vi "Coord window-Add to picture-Sel coord.vi"(6 "Value":i32[](array[numeric]), 7 "Feature to draw":enum16{"Draw point", "Draw square"}(ring), 9 "ItemNames":string[][](array[string]), 10 "new picture in":picture, 11 "Picture map ref in":refnum<vi>) -> (2 "new picture out":picture, 3 "Picture map ref":refnum<vi>)   [LabVIEW 2020]
panel:
  in  "color":u32(colorbox)=60927
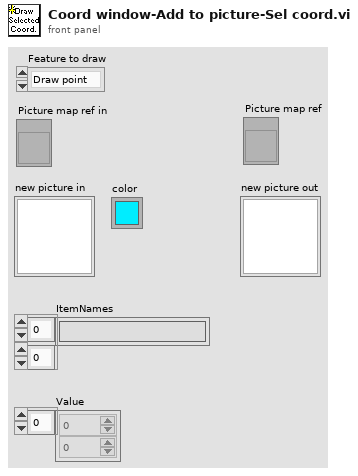
[diagram p1: front panel]
types:
  T1 = cluster{"Width":u16, "Style":enum32{"Solid", "Dash", "Dot", "DashDot", "DashDotDot"}}
  T2 = cluster{"Width":i16, "Style":enum32{"Solid", "Dash", "Dot", "DashDot", "DashDotDot"}}
  T3 = typedef "LVBoundsTypeDef.ctl" = cluster{"Width":u32, "Height":u32}
  T4 = cluster{"FOV/2-X (pixels)":i16, "FOV/2-Y (pixels)":i16}
  T5 = cluster{"left":i16, "top":i16, "right":i16, "bottom":i16}
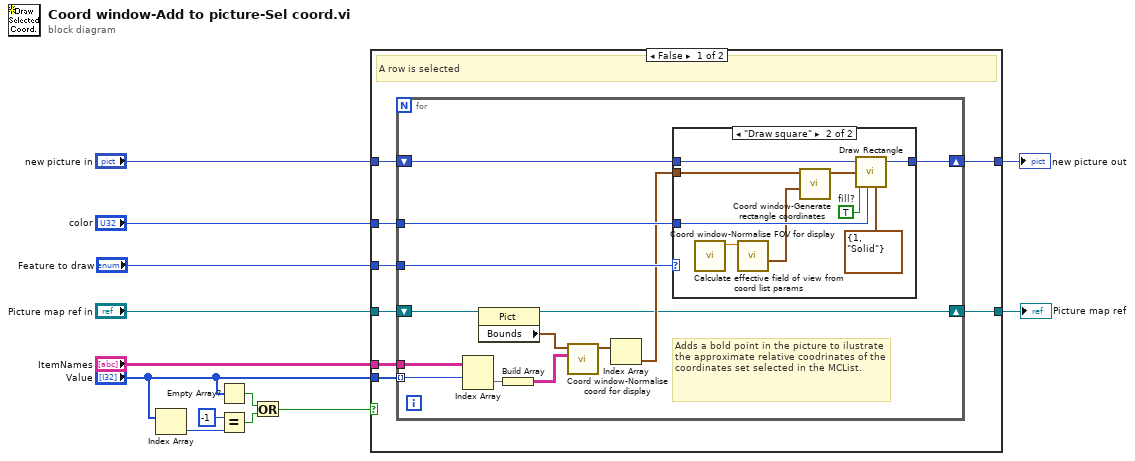
[diagram p0: block diagram]
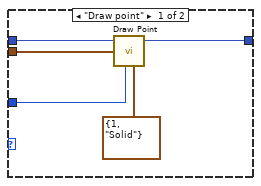
[diagram p2: hidden frame]
diagram:
  n1 = Index Array(array="Value") -> (element=w8:i32)  [unwired: 1 in]
  n2 = Empty Array?(array="Value") -> (empty?=w4:bool)
  n3 = Equal?(x=-1, y=w8) -> (x = y?=w5:bool)
  n4 = Or(x=w4, y=w5) -> (x .or. y?=w3:bool)
  n5 = case shown="False" w3 {
    tunnel: "new picture in" -> [w16 w50]
    tunnel: [w14 w50] -> w13
    tunnel: "Value" -> [w21 _]
    tunnel: "ItemNames" -> [w20 _]
    tunnel: "Picture map ref in" -> [w19 w49]
    tunnel: [w15 w49] -> w9
    tunnel: "color" -> [w17 _]
    tunnel: "Feature to draw" -> [w18 _]
    frame False {
      # "A row is selected"
      n6 = for {
        tunnel: w21 -> [w22] mode=indexing
        tunnel: w20 -> [w34]
        tunnel: w18 -> [w28]
        tunnel: w17 -> [w27]
        shift-right: [w24] -> w15
        shift-left: w19 -> [w30]
        shift-right: [w23] -> w14
        shift-left: w16 -> [w26]
        # "Adds a bold point in the picture to ilustrate the approximate relative coodrinates of the coordinates set selected in the MCList."
        n7 = Index Array(array=w34, index (row)=w22) -> (element=w33:string[])  [unwired: 1 in]
        n8 = property on="Property Node" class="Pict"(reference=w30) -> (reference out=w24:refnum<vi>, "Bounds"=w29:T3)  [unwired: 1 in, 1 out]
        n9 = Build Array(w33) -> (w32:string[][])
        n10 = call "Coord window-Normalise coord for display.vi"("MCList ItemNames"=w32, "Bounds"=w29) -> ("Normalised coordinates (for display)"=w31:cluster{"x":i16, "y":i16}[])  [unwired: 9 in]
        n11 = Index Array(array=w31) -> (element=w25:cluster{"x":i16, "y":i16})  [unwired: 1 in]
        n12 = case shown="\"Draw square\"" w28 {
          tunnel: w26 -> [w39 w48]
          tunnel: [w37 w47] -> w23
          tunnel: w25 -> [w36 w45]
          tunnel: w27 -> [w35 w46]
          frame "Draw point" {
            n13 = call <vilib>:"Draw Point.vi"("picture"=w39, "point(x,y)"=w36, "color(black)"=w35, "pen"=T1 {"Width"=1, "Style"=enum."Solid"}) -> ("new picture"=w37:picture)  [unwired: 5 in]
          }
          frame "Draw square" {
            w42 = TRUE  # fill?
            n14 = call "Calculate effective field of view from coord list params.vi"() -> ("Effective FOV (um)"=w40:sgl)  [unwired: 11 in]
            n15 = call "Coord window-Normalise FOV for display.vi"("Effective FOV (um)"=w40) -> ("Normalised Effective FOV/2"=w41:T4)  [unwired: 9 in, 1 out]
            n16 = call "Coord window-Generate rectangle coordinates.vi"("Normalised Effective FOV/2"=w41, "Norm point(x,y) (for display)"=w45) -> ("Norm rect (for display)"=w44:T5)  [unwired: 9 in]
            n17 = call <vilib>:"Draw Rectangle.vi"("picture"=w48, "rect"=w44, "fill?(F)"=w42, "color(black)"=w46, "pen"=T2 {"Width"=1, "Style"=enum."Solid"}) -> ("new picture"=w47:picture)  [unwired: 4 in]
          }
        }
      }
    }
    frame True {
      # "No row selected"
    }
  }
  "new picture out" <- w13
  "Picture map ref" <- w9
